vi "제목없음 9 (SubVI).vi"(0 "x":dbl, 1 "y":dbl, 2 "x 2":dbl, 3 "y 2":dbl) -> (7 "숫자형 컨트롤":dbl)   [LabVIEW 2018]
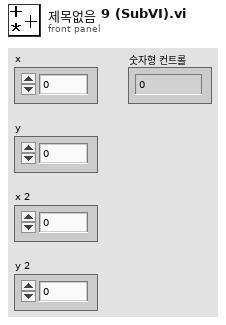
[diagram p1: front panel]
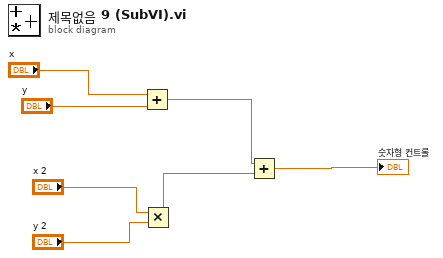
[diagram p0: block diagram]
diagram:
  n1 = Add(x="x", y="y") -> (x+y=w5:dbl)
  n2 = Multiply(x="x 2", y="y 2") -> (x*y=w6:dbl)
  n3 = Add(x=w5, y=w6) -> (x+y=→"숫자형 컨트롤":dbl)
